vi "Set Z Acceleration.vi"(8 "error in (no error)":errorcluster, 10 "mm/s":dbl=15.0 format="%#_13g", 11 "A3200 in":refnum<class "A3200.lvclass">) -> (0 "error out":errorcluster, 3 "A3200 out":refnum<class "A3200.lvclass">)   [LabVIEW 2016, in "A3200.lvclass"]
uses:
  A3200.lvclass
  Drivers/Aerotech A3200/Aerotech VIs.lvlib
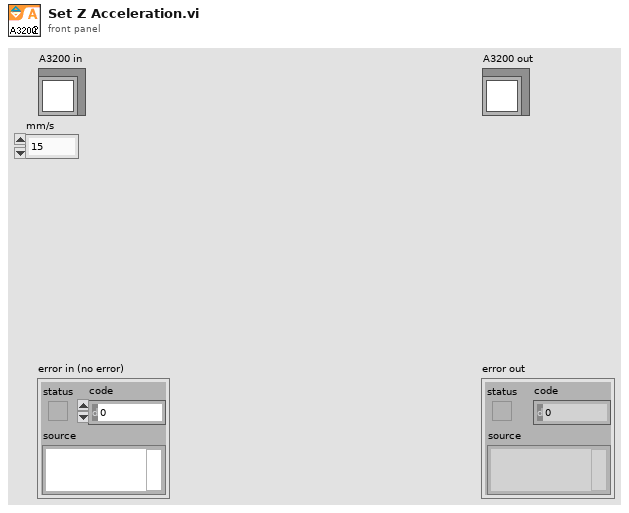
[diagram p1: front panel]
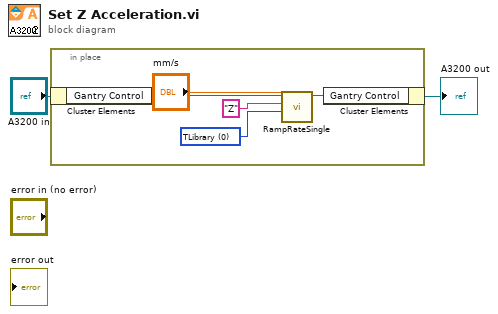
[diagram p0: block diagram]
diagram:
  n1 = in-place {
    w3 = 0 items=["TLibrary", "T01", "T02", "T03", "T04", "T05", "T06", "T07", "T08", "T09", "T10", "T11", "T12", "T13", "T14", "T15", "T16", "T17", "T18", "T19", "T20", "T21", "T22", "T23", "T24", "T25", "T26", "T27", "T28", "T29", "T30", "T31"] ("task id")
    n2 = in-place-cluster #1("A3200 in") -> ("Gantry Control"=w7:refnum<k24>)
    n3 = call "RampRateSingle.vi"("ramp rate"="mm/s", "task id"=w3, "axis name"="Z", "controller in"=w7) -> ("controller out"=w6:refnum<k24>)  [unwired: 6 in, 1 out]
    n4 = in-place-cluster #1("Gantry Control"=w6) -> (→"A3200 out":refnum<class "A3200.lvclass">)
  }
